vi "LJM_TCVoltsToTemp.vi"(7 "TCType":i32=6004, 8 "error in":errorcluster, 9 "CJTempK":dbl format="%.2f", 10 "TCVolts":dbl format="%.4f") -> (0 "error out":errorcluster, 1 "TCTempF":dbl format="%.2f", 2 "TCTempC":dbl format="%.2f", 3 "TCTempK":dbl format="%.2f")   [LabVIEW 2026]
uses:
  labjackm.dll
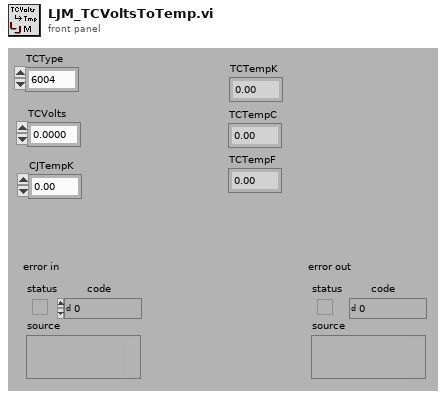
[diagram p1: front panel]
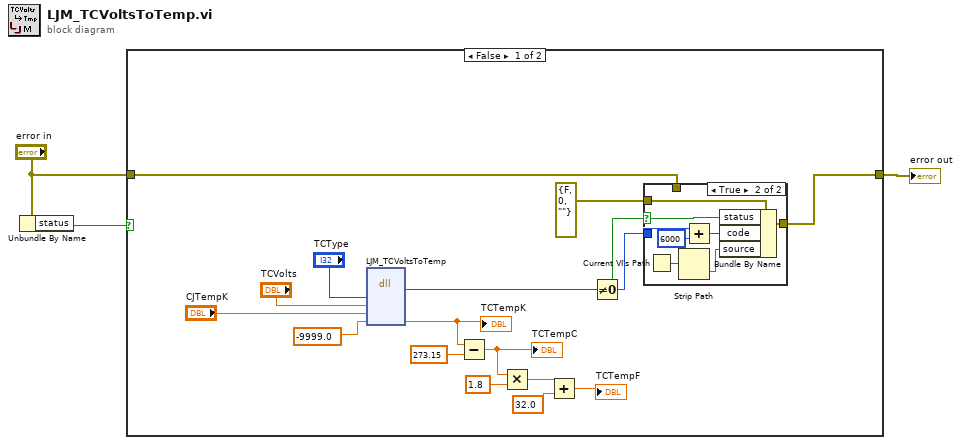
[diagram p0: block diagram]
diagram:
  n1 = Unbundle By Name("error in") -> ("status"=w3:bool)
  n2 = case shown="False" w3 {
    tunnel: "error in" -> [w16 w29]
    tunnel: [w15 w29] -> w1
    frame False {
      n3 = dll-call lib="labjackm.dll" fn="LJM_TCVoltsToTemp"("TCType"="TCType", "TCVolts"="TCVolts", "CJTempK"="CJTempK", "TCTempK"=-9999.0) -> (w19:i32, "TCTempK"=w10:dbl)  [unwired: 6 in, 2 out]
      "TCTempK" <- w10
      n4 = Subtract(x=w10, y=273.15) -> (x-y=w9:dbl)
      "TCTempC" <- w9
      n5 = Multiply(x=w9, y=1.8) -> (x*y=w14:dbl)
      n6 = Add(x=w14, y=32.0) -> (x+y=→"TCTempF":dbl)
      n7 = Not Equal To 0?(x=w19) -> (x != 0?=w18:bool)
      n8 = case shown="True" w18 {
        selector: w18 -> [_ w27]
        tunnel: [w20 w28] -> w15
        tunnel: errorcluster {"status"=FALSE, "code"=0, "source"=""} ("error IO") -> [_ w26]
        tunnel: w19 -> [_ w22]
        tunnel: w16 -> [w20 _]
        frame False {
        }
        frame True {
          n9 = Current VI's Path() -> (path=w24:path)
          n10 = Strip Path(path=w24) -> (name=w25:string)  [unwired: 1 out]
          n11 = Add(x=w22, y=6000) -> (x+y=w23:i32)
          n12 = Bundle By Name(cluster=w26, "status"=w27, "code"=w23, "source"=w25) -> (w28:errorcluster)
        }
      }
    }
    frame True {
    }
  }
  "error out" <- w1
